vi "FRIC_navX_Get_SystemInformation_Offsets.vi"(7 "Update":bool) -> (2 "Offsets":T1)   [LabVIEW 2015]
doc: "This navX VI returns the Offsets of the navX. This VI is rarely needed."
uses:
  navX Library v2/_TypeDefs/Z900_navX_DeviceRegisters.ctl
  navX Library v2/navX Library v2.lvlib
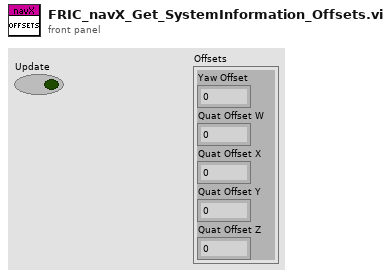
[diagram p1: front panel]
types:
  T1 = cluster{"Yaw Offset":dbl, "Quat Offset W":dbl, "Quat Offset X":dbl, "Quat Offset Y":dbl, "Quat Offset Z":dbl}
  T2 = typedef "navX Library v2.lvlib/Z900_navX_DeviceRegisters.ctl" = u8
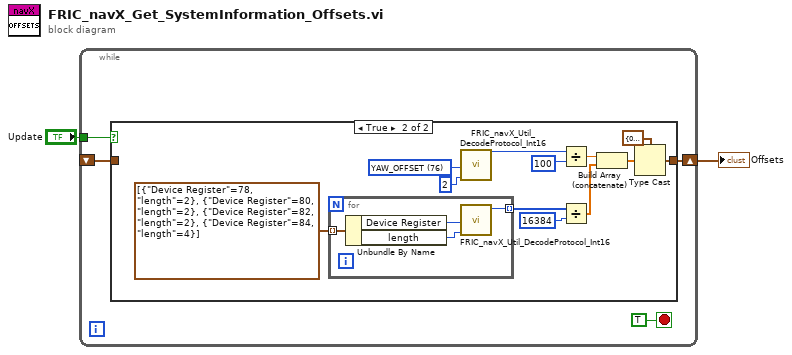
[diagram p0: block diagram]
diagram:
  n1 = while {
    shift-right: [w6] -> w2
    shift-left: _ -> [w3]
    tunnel: "Update" -> [w4]
    stop <- TRUE stop-if-true
    n2 = case shown="True" w4 {
      tunnel: [w7 w19] -> w6
      tunnel: w3 -> [w7 _]
      frame False {
      }
      frame True {
        w11 = T2 76 items=["WHOAMI"=0, "HW_REV"=1, "FW_VER_MAJOR"=2, "FW_VER_MINOR"=3, "UPDATE_RATE_HZ"=4, "ACCEL_FSR_G"=5, "GYRO_FSR_DPS"=6, "OP_STATUS"=8, "CAL_STATUS"=9, "SELFTEST_STATUS"=10, "CAPABILITY_FLAGS_L"=11, "CAPABILITY_FLAGS_H"=12, "SENSOR_STATUS"=16, "TIMESTAMP"=18, "YAW"=22, "ROLL"=24, "PITCH"=26, "HEADING"=28, "FUSED_HEADING"=30, "ALTITUDE_I"=32, "ALTITUDE_D"=34, "LINERA_ACC_X"=36, "LINERA_ACC_Y"=38, "LINERA_ACC_Z"=40, "QUAT_W"=42, "QUAT_X"=44, "QUAT_Y"=46, "QUAT_Z"=48, "MPU_TEMP_C"=50, "GYRO_X"=52, "GYRO_Y"=54, "GYRO_Z"=56, "ACC_X"=58, "ACC_Y"=60, "ACC_Z"=62, "MAG_X"=64, "MAG_Y"=66, "MAG_Z"=68, "PRESSURE_I"=70, "PRESSURE_D"=72, "PRESSURE_TEMP"=74, "YAW_OFFSET"=76, "QUAT_OFFSET_W"=78, "QUAT_OFFSET_X"=80, "QUAT_OFFSET_Y"=82, "QUAT_OFFSET_Z"=84, "INTEGRATION_CONTROL"=86, "VELOCITY_X"=88, "VELOCITY_Y"=92, "VELOCITY_Z"=96, "DISPLACMENT_X"=100, "DISPLACMENT_Y"=104, "DISPLACEMENT_Z"=108] ("Device Register")
        n3 = for {
          tunnel: cluster{"Device Register":T2, "length":i32}[] [{"Device Register"=78, "length"=2}, {"Device Register"=80, "length"=2}, {"Device Register"=82, "length"=2}, {"Device Register"=84, "length"=4}] ("Array") -> [w21] mode=indexing
          tunnel: [w20] -> w8 mode=indexing
          n4 = Unbundle By Name(w21) -> ("Device Register"=w23:T2, "length"=w22:i32)
          n5 = call "FRIC_navX_Util_DecodeProtocol_Int16.vi"("length"=w22, "Device Register"=w23) -> ("Value"=w20:i16)  [unwired: 9 in]
        }
        n6 = call "FRIC_navX_Util_DecodeProtocol_Int16.vi"("length"=2, "Device Register"=w11) -> ("Value"=w12:i16)  [unwired: 9 in]
        n7 = Divide(x=w12, y=100) -> (x/y=w15:dbl)
        n8 = Divide(x=w8, y=u16 16384) -> (x/y=w13:dbl[])
        n9 = Build Array (concatenate)(w15, w13) -> (w18:dbl[])
        n10 = Type Cast(type=T1 {"Yaw Offset"=0.0, "Quat Offset W"=0.0, "Quat Offset X"=0.0, "Quat Offset Y"=0.0, "Quat Offset Z"=0.0}, x=w18) -> (*(type *) &x=w19:T1)
      }
    }
  }
  "Offsets" <- w2
